vi "Read lRMS_hw.vi"(8 "error in (no error)":errorcluster, 11 "cPAS Cell in":refnum<class "cPAS Cell Data.lvclass">) -> (0 "error out":errorcluster, 2 "lRMS_hw":sgl, 3 "cPAS Cell out":refnum<class "cPAS Cell Data.lvclass">)   [LabVIEW 2015, in "cPAS Cell Data.lvclass"]
uses:
  cPAS Cell Data.lvclass
  cPAS Cell Data.lvclass/cPAS Cell Data.ctl
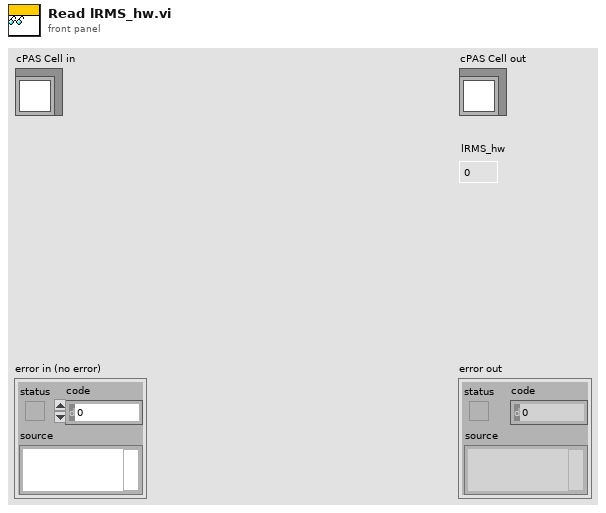
[diagram p1: front panel]
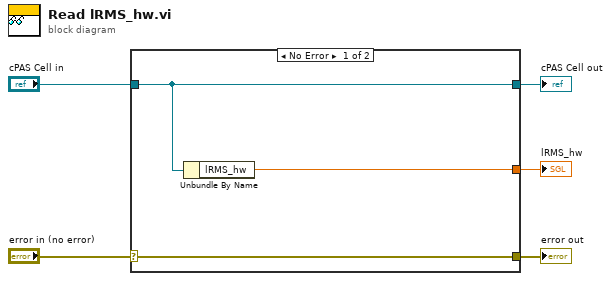
[diagram p0: block diagram]
diagram:
  n1 = case shown="No Error" "error in (no error)" {
    selector: "error in (no error)" -> [w8 w9]
    tunnel: [w8 w9] -> w4
    tunnel: [w7 w10] -> w2
    tunnel: "cPAS Cell in" -> [w7 w10]
    tunnel: [w6 _] -> w1
    frame No Error {
      n2 = Unbundle By Name(w7) -> ("lRMS_hw"=w6:sgl)
    }
    frame Error {
    }
  }
  "error out" <- w4
  "cPAS Cell out" <- w2
  "lRMS_hw" <- w1
